vi "E4_Taladro.vi"() -> ()   [LabVIEW 2024]
panel:
  in  "PARO":bool
  out "Gruesas":i32
  out "Delgadas":i32
  out "A3":bool
  in  "Pieza Gruesa":bool
  in  "Inicio":bool
  in  "?":bool
  out "A0":bool
  out "A1":bool
  out "A2":bool
  # "Pieza Delgada"
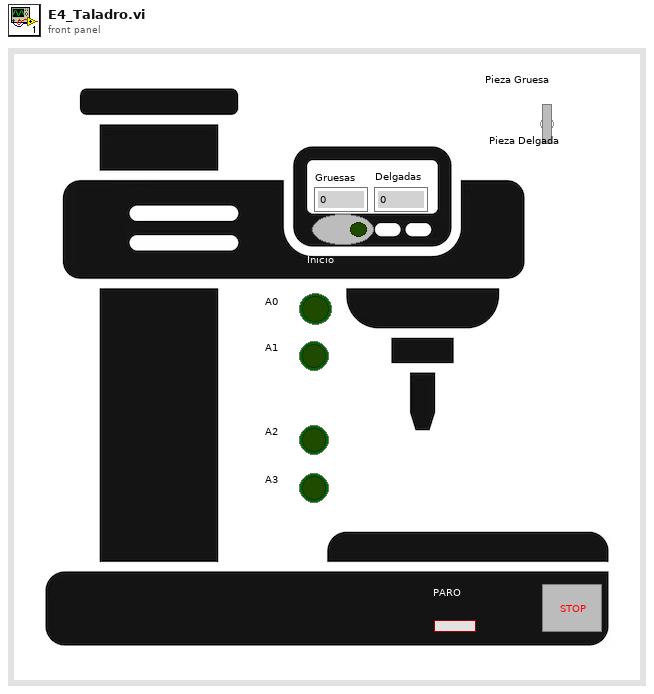
[diagram p1: front panel]
types:
  T1 = enum16{"EstadoDefecto", "Estado1", "Estado2", "Estado3", "Estado4", "Estado5", "Estado6", "Estado7", "Estado8", "Estado9"}
  T2 = enum16{"EstadoDefecto", "Estado1", "Estado2", "Estado3", "Estado4", "Estado5", "Estado6"}
  T3 = enum16{"EstadoDefecto", "Estado1", "Estado2", "Estado3", "Estado4", "Estado5", "Estado6", "Estado7"}
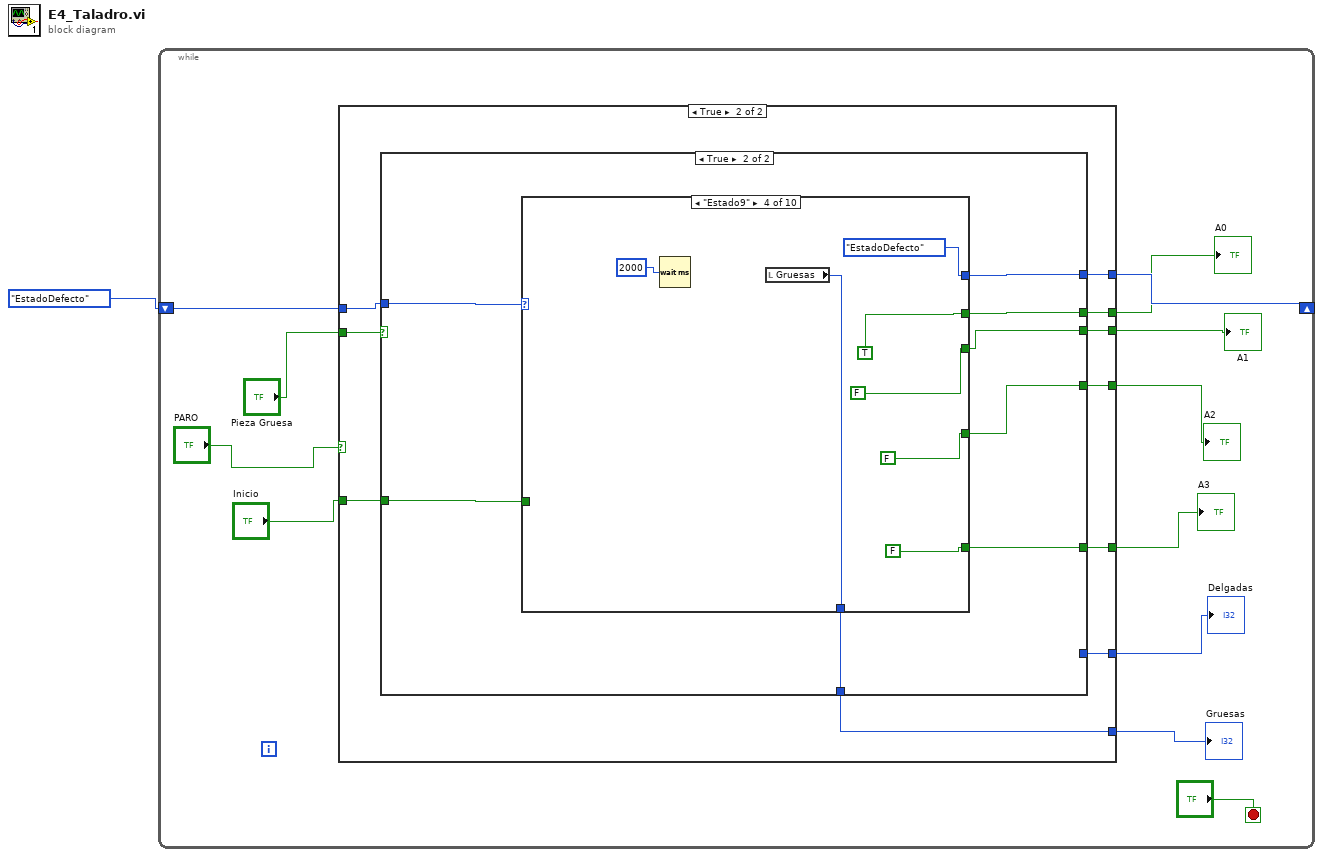
[diagram p0: block diagram]
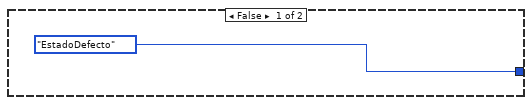
[diagram p2: hidden frame]
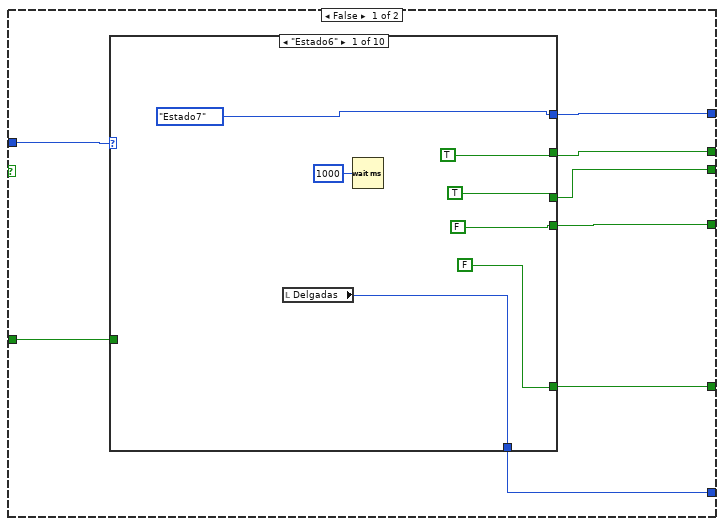
[diagram p3: hidden frame]
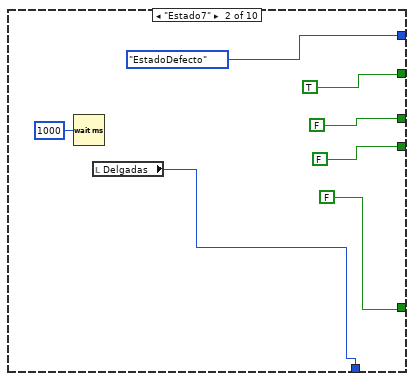
[diagram p4: hidden frame]
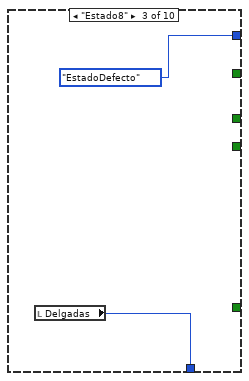
[diagram p5: hidden frame]
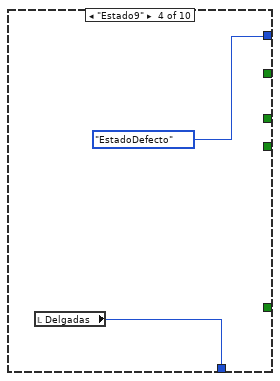
[diagram p6: hidden frame]
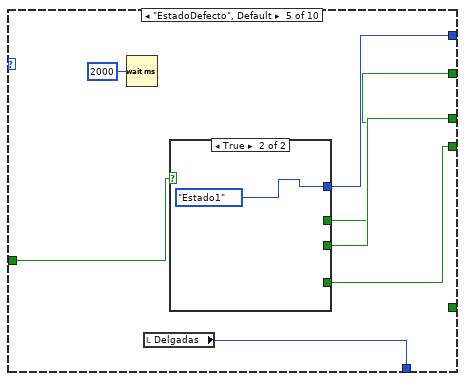
[diagram p7: hidden frame]
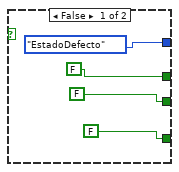
[diagram p8: hidden frame]
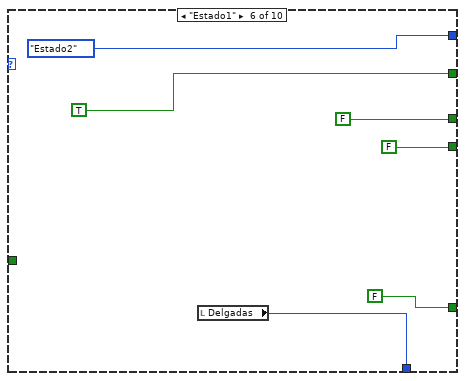
[diagram p9: hidden frame]
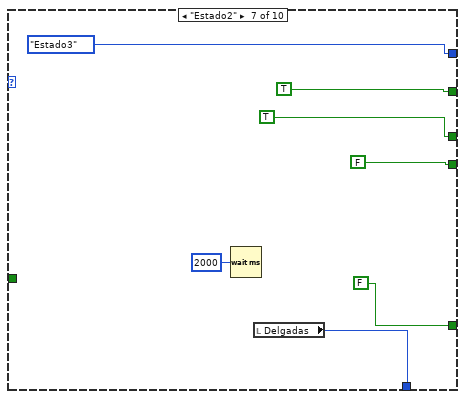
[diagram p10: hidden frame]
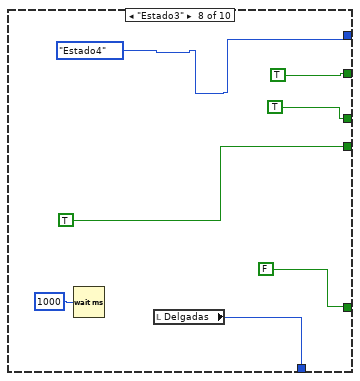
[diagram p11: hidden frame]
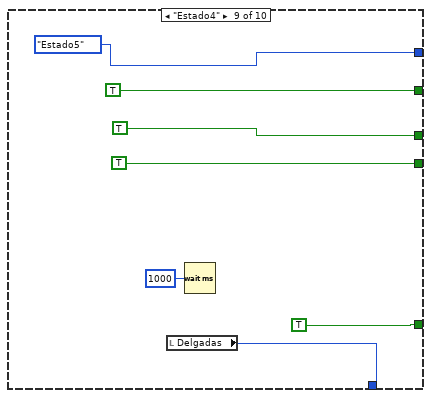
[diagram p12: hidden frame]
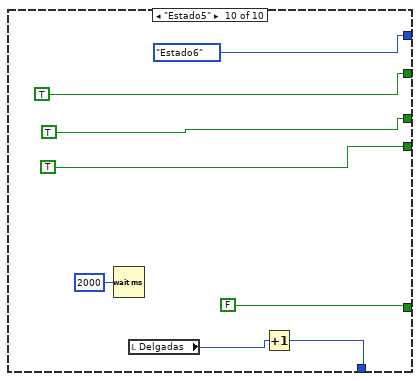
[diagram p13: hidden frame]
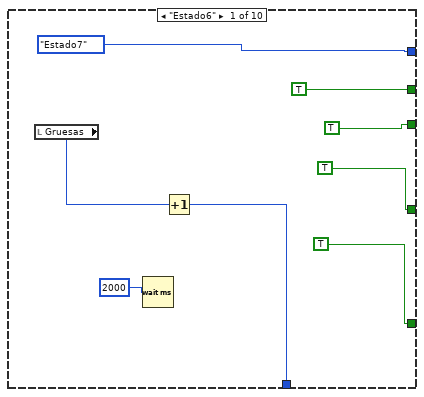
[diagram p14: hidden frame]
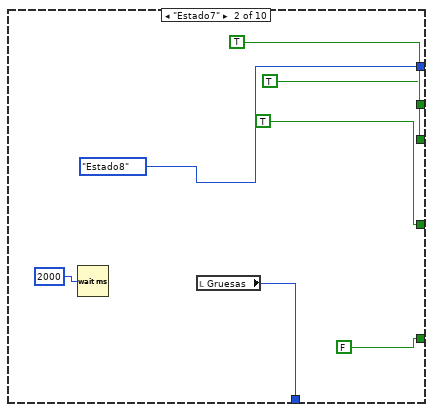
[diagram p15: hidden frame]
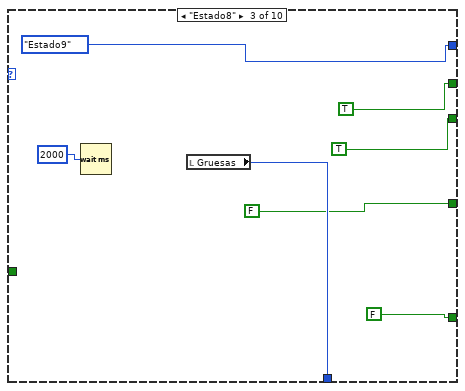
[diagram p16: hidden frame]
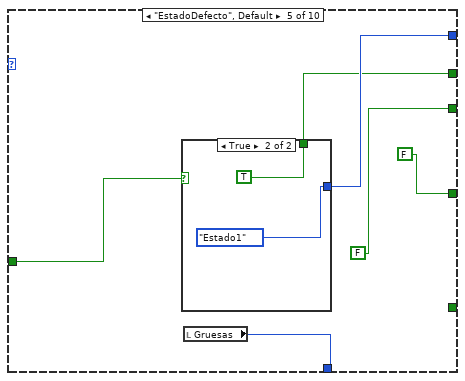
[diagram p17: hidden frame]
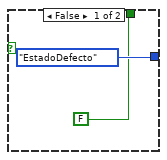
[diagram p18: hidden frame]
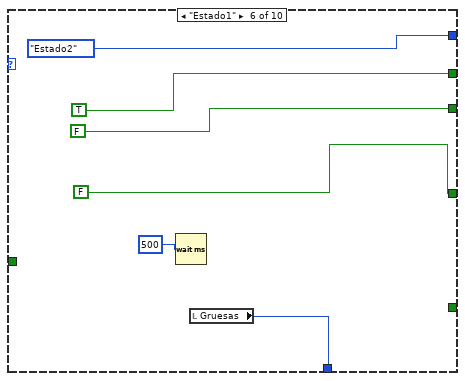
[diagram p19: hidden frame]
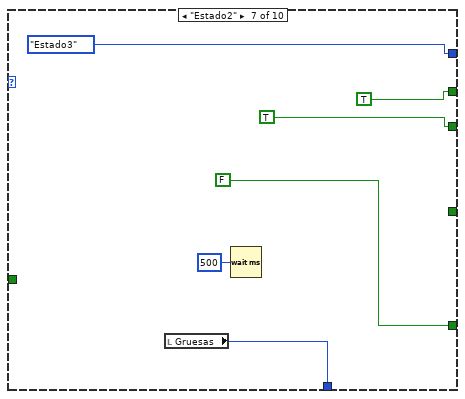
[diagram p20: hidden frame]
diagram:
  n1 = while {
    shift-right: [w11] -> _
    shift-left: T1."EstadoDefecto" -> [w12]
    stop <- "?" stop-if-true
    n2 = case shown="True" "PARO" {
      tunnel: w12 -> [_ w24]
      tunnel: [T1."EstadoDefecto" w23] -> w11
      tunnel: [_ w22] -> w10
      tunnel: [_ w21] -> w9
      tunnel: [_ w20] -> w8
      tunnel: "Pieza Gruesa" -> [_ w19]
      tunnel: "Inicio" -> [_ w18]
      tunnel: [_ w17] -> w5
      tunnel: [_ w16] -> w4
      tunnel: [_ w15] -> w3
      frame False {
      }
      frame True {
        n3 = case shown="True" w19 {
          tunnel: w24 -> [w28 w105]
          tunnel: [w29 w104] -> w23
          tunnel: [w30 w103] -> w22
          tunnel: [w31 w102] -> w21
          tunnel: [w32 w101] -> w20
          tunnel: w18 -> [w27 w100]
          tunnel: [w26 w99] -> w17
          tunnel: [_ w98] -> w16
          tunnel: [w25 _] -> w15
          frame False {
            n4 = case shown="\"Estado6\"" w28 {
              tunnel: [T1."Estado7" T2."EstadoDefecto" T2."EstadoDefecto" T2."EstadoDefecto" w57 T2."Estado2" T2."Estado3" T2."Estado4" T2."Estado5" T2."Estado6"] -> w29
              tunnel: [TRUE TRUE _ _ w53 TRUE TRUE TRUE TRUE TRUE] -> w30
              tunnel: [TRUE FALSE _ _ w55 FALSE TRUE TRUE TRUE TRUE] -> w31
              tunnel: [FALSE FALSE _ _ w54 FALSE FALSE TRUE TRUE TRUE] -> w32
              tunnel: [FALSE FALSE _ _ _ FALSE FALSE FALSE TRUE FALSE] -> w26
              tunnel: w27 -> [_ _ _ _ w56 _ _ _ _ _]
              tunnel: [w38 w45 w47 w49 w51 w66 w71 w77 w83 w90] -> w25
              frame "Estado6" {
                n5 = local read "Delgadas"() -> (w38:i32)
                n6 = Wait (ms)(milliseconds to wait=u32 1000) -> ()  [unwired: 1 out]
              }
              frame "Estado7" {
                n7 = Wait (ms)(milliseconds to wait=u32 1000) -> ()  [unwired: 1 out]
                n8 = local read "Delgadas"() -> (w45:i32)
              }
              frame "Estado8" {
                n9 = local read "Delgadas"() -> (w47:i32)
              }
              frame "Estado9" {
                n10 = local read "Delgadas"() -> (w49:i32)
              }
              frame "EstadoDefecto", Default {
                n11 = Wait (ms)(milliseconds to wait=u32 2000) -> ()  [unwired: 1 out]
                n12 = local read "Delgadas"() -> (w51:i32)
                n13 = case shown="True" w56 {
                  tunnel: [T2."EstadoDefecto" T2."Estado1"] -> w57
                  tunnel: [FALSE _] -> w55
                  tunnel: [FALSE _] -> w54
                  tunnel: [FALSE _] -> w53
                  frame False {
                  }
                  frame True {
                  }
                }
              }
              frame "Estado1" {
                n14 = local read "Delgadas"() -> (w66:i32)
              }
              frame "Estado2" {
                n15 = Wait (ms)(milliseconds to wait=u32 2000) -> ()  [unwired: 1 out]
                n16 = local read "Delgadas"() -> (w71:i32)
              }
              frame "Estado3" {
                n17 = Wait (ms)(milliseconds to wait=u32 1000) -> ()  [unwired: 1 out]
                n18 = local read "Delgadas"() -> (w77:i32)
              }
              frame "Estado4" {
                n19 = local read "Delgadas"() -> (w83:i32)
                n20 = Wait (ms)(milliseconds to wait=u32 1000) -> ()  [unwired: 1 out]
              }
              frame "Estado5" {
                n21 = Wait (ms)(milliseconds to wait=u32 2000) -> ()  [unwired: 1 out]
                n22 = local read "Delgadas"() -> (w91:i32)
                n23 = Increment(x=w91) -> (x+1=w90:i32)
              }
            }
          }
          frame True {
            n24 = case shown="\"Estado9\"" w105 {
              tunnel: [T3."Estado7" T1."Estado8" T1."Estado9" T1."EstadoDefecto" w139 T2."Estado2" T2."Estado3" T2."Estado4" T2."Estado5" T2."Estado6"] -> w104
              tunnel: [TRUE TRUE TRUE TRUE w135 TRUE TRUE TRUE TRUE TRUE] -> w103
              tunnel: [TRUE TRUE TRUE FALSE FALSE FALSE TRUE TRUE TRUE TRUE] -> w102
              tunnel: [TRUE TRUE FALSE FALSE FALSE FALSE _ TRUE FALSE TRUE] -> w101
              tunnel: w100 -> [_ _ _ _ w140 _ _ _ _ _]
              tunnel: [TRUE FALSE FALSE FALSE _ _ FALSE FALSE _ _] -> w99
              tunnel: [w108 w115 w126 w132 w136 w146 w151 w157 w164 w170] -> w98
              frame "Estado6" {
                n25 = local read "Gruesas"() -> (w107:i32)
                n26 = Wait (ms)(milliseconds to wait=u32 2000 ("y")) -> ()  [unwired: 1 out]
                n27 = Increment(x=w107) -> (x+1=w108:i32)
              }
              frame "Estado7" {
                n28 = Wait (ms)(milliseconds to wait=u32 2000 ("y")) -> ()  [unwired: 1 out]
                n29 = local read "Gruesas"() -> (w115:i32)
              }
              frame "Estado8" {
                n30 = Wait (ms)(milliseconds to wait=u32 2000 ("y")) -> ()  [unwired: 1 out]
                n31 = local read "Gruesas"() -> (w126:i32)
              }
              frame "Estado9" {
                n32 = Wait (ms)(milliseconds to wait=u32 2000 ("y")) -> ()  [unwired: 1 out]
                n33 = local read "Gruesas"() -> (w132:i32)
              }
              frame "EstadoDefecto", Default {
                n34 = case shown="True" w140 {
                  tunnel: [T2."EstadoDefecto" T2."Estado1"] -> w139
                  tunnel: [FALSE TRUE] -> w135
                  frame False {
                  }
                  frame True {
                  }
                }
                n35 = local read "Gruesas"() -> (w136:i32)
              }
              frame "Estado1" {
                n36 = Wait (ms)(milliseconds to wait=u32 500 ("y")) -> ()  [unwired: 1 out]
                n37 = local read "Gruesas"() -> (w146:i32)
              }
              frame "Estado2" {
                n38 = local read "Gruesas"() -> (w151:i32)
                n39 = Wait (ms)(milliseconds to wait=u32 500) -> ()  [unwired: 1 out]
              }
              frame "Estado3" {
                n40 = local read "Gruesas"() -> (w157:i32)
                n41 = Wait (ms)(milliseconds to wait=u32 2000 ("y")) -> ()  [unwired: 1 out]
              }
              frame "Estado4" {
                n42 = Wait (ms)(milliseconds to wait=u32 2000 ("y")) -> ()  [unwired: 1 out]
                n43 = local read "Gruesas"() -> (w164:i32)
              }
              frame "Estado5" {
                n44 = local read "Gruesas"() -> (w170:i32)
                n45 = Wait (ms)(milliseconds to wait=u32 2000 ("y")) -> ()  [unwired: 1 out]
              }
            }
          }
        }
      }
    }
    "A0" <- w10
    "A1" <- w9
    "A2" <- w8
    "A3" <- w5
    "Delgadas" <- w3
    "Gruesas" <- w4
  }
